vi "PDLM_GetLHTargetTempLimits.vi"(8 "error in (no error)":errorcluster, 10 "ScaleID":T1, 11 "USBIdx":i32) -> (0 "error out":errorcluster, 1 "MaxTemp":sgl, 2 "MinTemp":sgl, 3 "return type":i32)   [LabVIEW 2017]
uses:
  PDLM_ScaleID.ctl
  PDLM_DllPath_global.vi
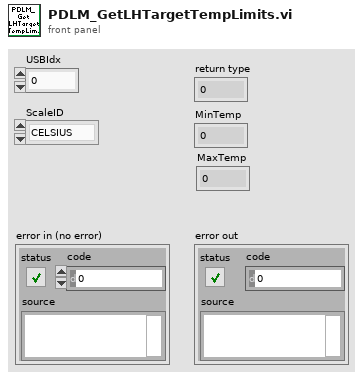
[diagram p1: front panel]
types:
  T1 = typedef "PDLM_ScaleID.ctl" = enum32{"CELSIUS", "FAHRENHEIT", "KELVIN"}
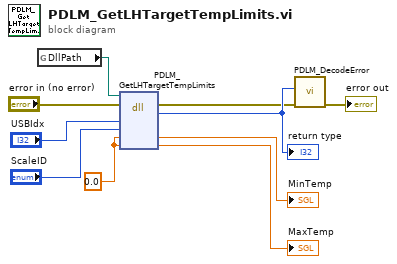
[diagram p0: block diagram]
diagram:
  w2 = sgl 0.0 ("mode")
  n1 = global read "PDLM_DllPath_global.vi" "DllPath"() -> (w6:path)
  n2 = dll-call lib="M:/_dev/progs/LabVIEW/_lib/PQ/Taiko/pdlm_lib.dll" fn="PDLM_GetLHTargetTempLimits"(path in=w6, error in="error in (no error)", "USBIdx"="USBIdx", "ScaleID"="ScaleID", "MinTemp"=w2, "MaxTemp"=w2) -> (error out=w8:errorcluster, "return type"=w9:i32, "MinTemp"=→"MinTemp":sgl, "MaxTemp"=→"MaxTemp":sgl)  [unwired: 3 in, 1 out]
  "return type" <- w9
  n3 = call "PDLM_DecodeError.vi"("error in (no error)"=w8, "code"=w9) -> ("error out"=→"error out":errorcluster)  [unwired: 7 in, 2 out]
